vi "ColorMeasurement.vi"() -> (0 "CLEAR INPUT":dynamicdata(waveform), 1 "GREEN INPUT":dynamicdata(waveform), 2 "CLEAR Frequency":dbl, 3 "GREEN Frequency":dbl, 4 "BLUE INPUT":dynamicdata(waveform), 5 "RED Frequency":dbl, 6 "RED INPUT":dynamicdata(waveform), 7 "BLUE Frequency":dbl)   [LabVIEW 2022 SP3]
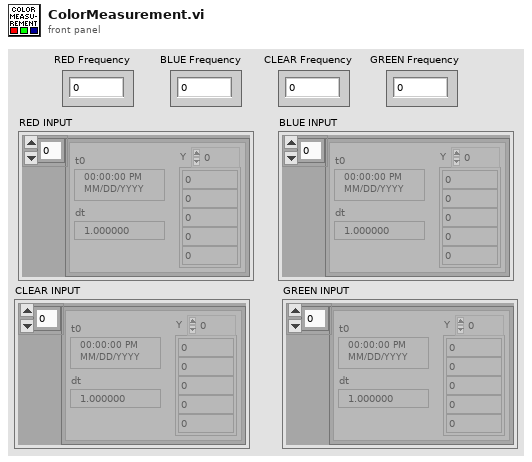
[diagram p1: front panel]
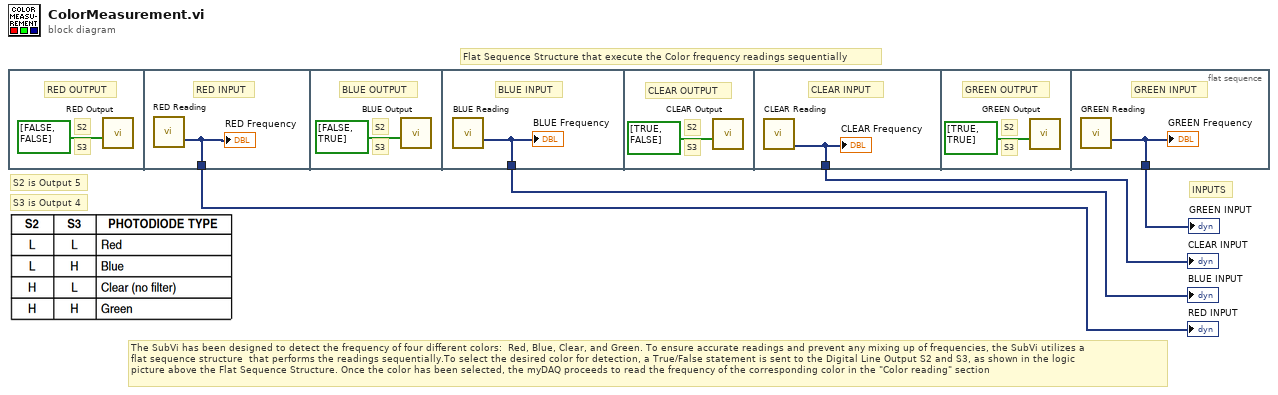
[diagram p0: block diagram]
diagram:
  # "The SubVi has been designed to detect the frequency of four different colors:  Red, Blue, Clear, and Green. To ensure accurate readings and prevent any mixing up of frequencies, the SubVi utilizes a \nflat sequence structure  that performs the readings sequentially.To select the desired color for detection, a True/False statement is sent to the Digital Line Output S2 and S3, as shown in the logic\npicture above the Flat Sequence Structure. Once the color has been selected, the myDAQ proceeds to read the frequency of the corresponding color in the \"Color reading\" section"
  # "INPUTS"
  # "Flat Sequence Structure that execute the Color frequency readings sequentially"
  # "S3 is Output 4"
  # "S2 is Output 5"
  n1 = flat-sequence {
    tunnel: [w6] -> w2
    tunnel: [w8] -> w4
    tunnel: [w10] -> w3
    tunnel: [w12] -> w1
    frame #0 {
      # "S3"
      # "S2"
      # "RED OUTPUT"
      n2 = call "RED Output"("data"=bool[] [FALSE, FALSE]) -> ()  [unwired: 17 in, 2 out]
    }
    frame #1 {
      # "RED INPUT"
      n3 = call "RED Reading"() -> ("data"=w6:dynamicdata)  [unwired: 17 in, 2 out]
      "RED Frequency" <- w6
    }
    frame #2 {
      # "S3"
      # "S2"
      # "BLUE OUTPUT"
      n4 = call "BLUE Output"("data"=bool[] [FALSE, TRUE]) -> ()  [unwired: 17 in, 2 out]
    }
    frame #3 {
      # "BLUE INPUT"
      n5 = call "BLUE Reading"() -> ("data"=w8:dynamicdata)  [unwired: 17 in, 2 out]
      "BLUE Frequency" <- w8
    }
    frame #4 {
      # "S3"
      # "S2"
      # "CLEAR OUTPUT"
      n6 = call "CLEAR Output"("data"=bool[] [TRUE, FALSE]) -> ()  [unwired: 17 in, 2 out]
    }
    frame #5 {
      # "CLEAR INPUT"
      n7 = call "CLEAR Reading"() -> ("data"=w10:dynamicdata)  [unwired: 17 in, 2 out]
      "CLEAR Frequency" <- w10
    }
    frame #6 {
      # "S3"
      # "S2"
      # "GREEN OUTPUT"
      n8 = call "GREEN Output"("data"=bool[] [TRUE, TRUE]) -> ()  [unwired: 17 in, 2 out]
    }
    frame #7 {
      # "GREEN INPUT"
      n9 = call "GREEN Reading"() -> ("data"=w12:dynamicdata)  [unwired: 17 in, 2 out]
      "GREEN Frequency" <- w12
    }
  }
  "BLUE INPUT" <- w4
  "GREEN INPUT" <- w1
  "CLEAR INPUT" <- w3
  "RED INPUT" <- w2
